vi "IMAQdx LL-Grab Raw Data.vi"(8 "ErrIn":errorcluster, 11 "Camera":refnum<k21> caption="IMAQdx Session") -> (0 "ErrOut":errorcluster)   [LabVIEW 2013]
doc: "Use this template to build a VI to use as a subVI."
uses:
  <vilib>/vision/driver/IMAQdx.llb/IMAQdx Acquisition Mode.ctl
  <vilib>/vision/driver/IMAQdx.llb/IMAQdx Buffer Number Mode.ctl
  <vilib>/vision/driver/NI_Vision_Acquisition_Software.lvlib
panel:
  out "Image Data Array":u8[](array[numeric])
  in  "stop":bool
  out "Frame Rate":dbl
  # "Input Parameters"
  # "Output Parameters"
  # "VI Description:\nThis VI is created to snap a image from imaging device."
  # ":: MVI Framework V1.0 ::\nAuthor:Gaoke Yang\nEmail: gaoke.yang@yahoo.com\nWeb: www.mvicontrol.com\nCopyright (C) 2013, MVI Technologies All Rights Reserved"
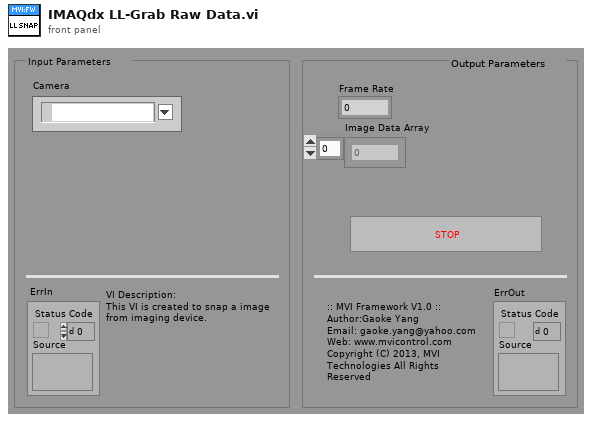
[diagram p1: front panel]
types:
  T1 = typedef "NI_Vision_Acquisition_Software.lvlib/IMAQdx Acquisition Mode.ctl" = enum32{"One Shot", "Continuous"}
  T2 = typedef "IMAQdx.ctl" = refnum<k21>
  T3 = typedef "NI_Vision_Acquisition_Software.lvlib/IMAQdx Buffer Number Mode.ctl" = enum32{"Next", "Last", "Buffer Number"}
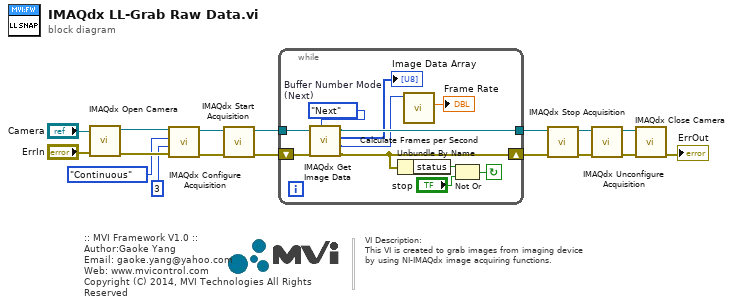
[diagram p0: block diagram]
diagram:
  # "VI Description:\nThis VI is created to grab images from imaging device \nby using NI-IMAQdx image acquiring functions."
  # ":: MVI Framework V1.0 ::\nAuthor:Gaoke Yang\nEmail: gaoke.yang@yahoo.com\nWeb: www.mvicontrol.com\nCopyright (C) 2014, MVI Technologies All Rights Reserved"
  n1 = call <vilib>:"IMAQdx Open Camera.vi"("error in"="ErrIn", "Session In"="Camera") -> ("error out"=w13:errorcluster, "Session Out"=w14:T2)  [unwired: 8 in]
  n2 = call <vilib>:"IMAQdx Configure Acquisition.vi"("error in"=w13, "Number of Buffers"=u32 3, "Continuous?"=IMAQdx_Acquisition_Mode."Continuous", "Session In"=w14) -> ("error out"=w2:errorcluster, "Session Out"=w10:T2)  [unwired: 6 in]
  n3 = call <vilib>:"IMAQdx Start Acquisition.vi"("error in"=w2, "Session In"=w10) -> ("error out"=w8:errorcluster, "Session Out"=w9:T2)  [unwired: 8 in]
  n4 = while {
    shift-left: w8 -> [w23]
    shift-right: [w19] -> w6
    tunnel: w9 -> [w24]
    tunnel: [w21] -> w5
    stop <- w27 continue-if-true
    w22 = IMAQdx_Buffer_Number_Mode."Next"  # Buffer Number Mode (Next)
    n5 = call <vilib>:"IMAQdx Get Image Data.vi"("Buffer Number Mode (Next)"=w22, "error in"=w23, "Session In"=w24) -> ("error out"=w19:errorcluster, "Buffer Number Out"=w20:u32, "Image Data Array"=→"Image Data Array":u8[], "Session Out"=w21:T2)  [unwired: 1 in, 4 out]
    n6 = Unbundle By Name(w19) -> ("status"=w25:bool)
    n7 = call <vilib>:"Calculate Frames per Second.vi"("Buffer Number"=w20) -> ("Processed Frames/s"=→"Frame Rate":dbl)  [unwired: 8 in, 2 out]
    n8 = Not Or(1:"stop", 2:w25) -> (0:w27:bool)
  }
  n9 = call <vilib>:"IMAQdx Stop Acquisition.vi"("error in"=w6, "Session In"=w5) -> ("error out"=w4:errorcluster, "Session Out"=w16:T2)  [unwired: 8 out]
  n10 = call <vilib>:"IMAQdx Unconfigure Acquisition.vi"("error in"=w4, "Session In"=w16) -> ("error out"=w3:errorcluster, "Session Out"=w17:T2)  [unwired: 8 out]
  n11 = call <vilib>:"IMAQdx Close Camera.vi"("error in"=w3, "Session In"=w17) -> ("error out"=→"ErrOut":errorcluster)  [unwired: 9 out]
